vi "Splash Screen.vi"(8 "error in (no error)":errorcluster, 11 "Start Splash Screen":bool) -> (0 "error out":errorcluster)   [LabVIEW 2023]
uses:
  Type Definitions/UTILITY Notifier.ctl
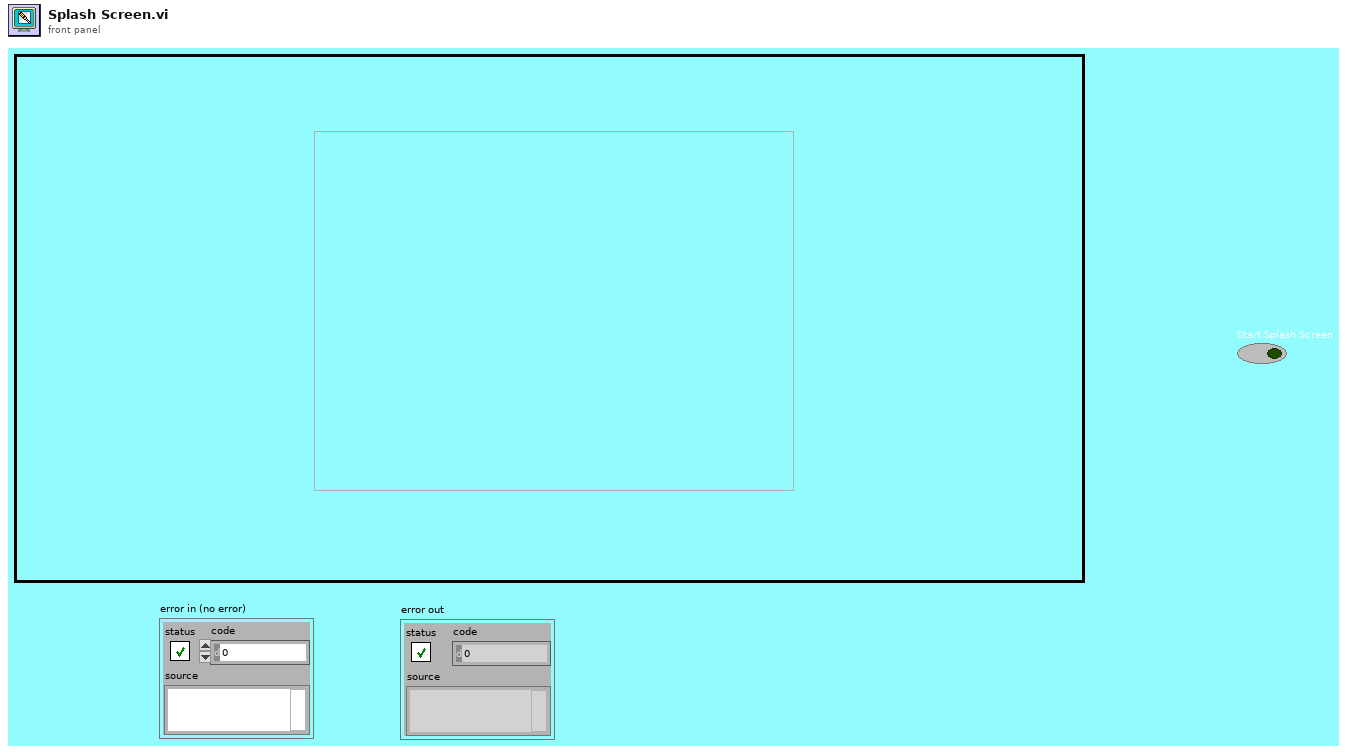
[diagram p1: front panel]
types:
  T1 = typedef "UTILITY Notifier.ctl" = enum16{"Set", "Read", "Release Ref"}
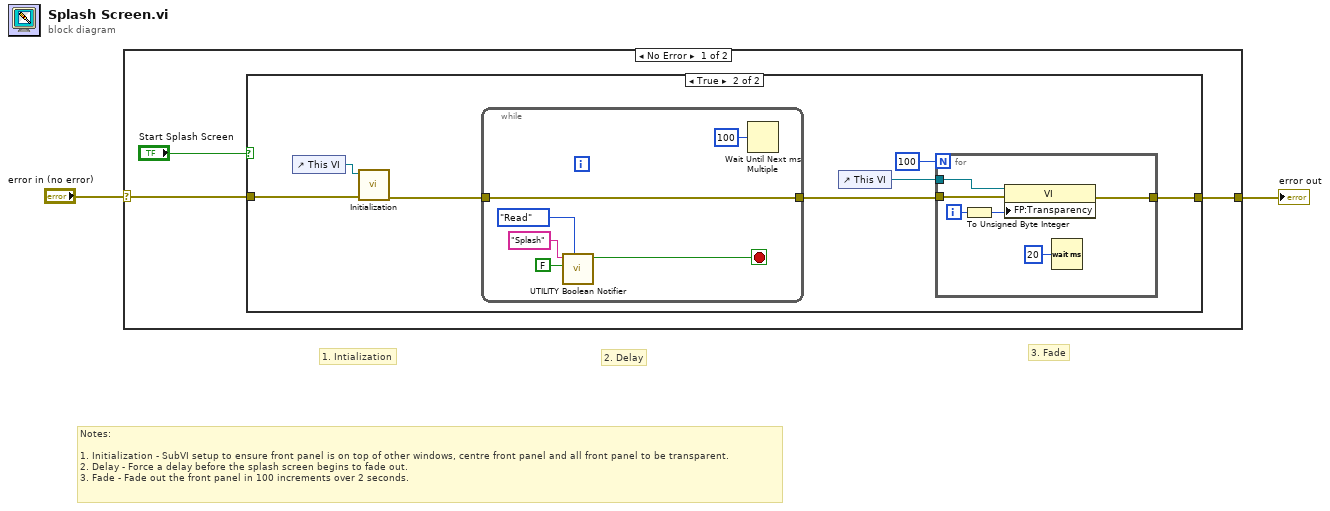
[diagram p0: block diagram]
diagram:
  # "Notes:\n\n1. Initialization - SubVI setup to ensure front panel is on top of other windows, centre front panel and all front panel to be transparent.\n2. Delay - Force a delay before the splash screen begins to fade out.\n3. Fade - Fade out the front panel in 100 increments over 2 seconds."
  # "3. Fade"
  # "2. Delay"
  # "1. Intialization"
  n1 = case shown="No Error" "error in (no error)" {
    selector: "error in (no error)" -> [w4 w26]
    tunnel: [w5 w26] -> w2
    frame No Error {
      n2 = case shown="True" "Start Splash Screen" {
        tunnel: [w6 w12] -> w5
        tunnel: w4 -> [w6 w10]
        frame False {
        }
        frame True {
          n3 = control-ref of="This VI"() -> (w9:refnum<vi>)
          n4 = call "Initialization.vi"("error in"=w10, "VI Refnum"=w9) -> ("error out"=w8:errorcluster)  [unwired: 9 in]
          n5 = while {
            tunnel: w8 -> [w18]
            tunnel: [w18] -> w7
            stop <- w14 stop-if-true
            n6 = call "UTILITY Boolean Notifier.vi"("Status"=UTILITY_Notifier."Read", "Set Status"=FALSE, "name (unnamed)"="Splash") -> ("latest READ notification"=w14:bool)  [unwired: 7 in, 1 out]
            n7 = Wait Until Next ms Multiple(millisecond multiple=u32 100) -> ()  [unwired: 1 out]
          }
          n8 = control-ref of="This VI"() -> (w11:refnum<vi>)
          n9 = for {
            N: 100 -> [_]
            tunnel: [w23] -> w12
            tunnel: w11 -> [w21]
            tunnel: w7 -> [w20]
            i -> [w25]
            n10 = To Unsigned Byte Integer(number=w25) -> (unsigned 8bit integer=w24:u8)
            n11 = property class="VI"(reference=w21, error in=w20, "FP:Transparency"=w24) -> (error out=w23:errorcluster)  [unwired: 1 out]
            n12 = Wait (ms)(milliseconds to wait=u32 20) -> ()  [unwired: 1 out]
          }
        }
      }
    }
    frame Error {
    }
  }
  "error out" <- w2
